vi "YKMW100 Write Com Register.vi"(0 "VISA session":refnum<visa-resource-name>="MW100", 2 "Semiphore":T1, 5 "Channel":string="C001", 7 "Value":string="000", 11 "error in (no error)":errorcluster) -> (4 "dup VISA session":refnum<visa-resource-name>="MW100", 15 "error out":errorcluster)   [LabVIEW 2009]
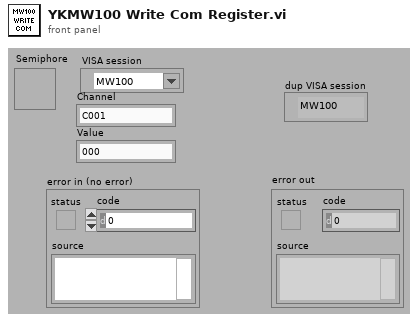
[diagram p1: front panel]
types:
  T1 = typedef "Semaphore RefNum" = refnum<k1>
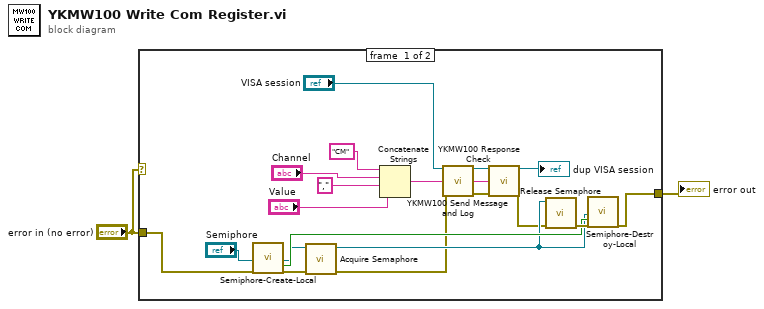
[diagram p0: block diagram]
diagram:
  n1 = case shown="No Error" "error in (no error)" {
    selector: "error in (no error)" -> [_ w23]
    tunnel: [w5 w23] -> w2
    tunnel: "error in (no error)" -> [w6 _]
    frame #0 {
      n2 = call "Semiphore-Create-Local.vi"("Semiphore"="Semiphore", "error in (no error)"=w6) -> ("semaphore"=w8:T1, "Local?"=w11:bool, "error out"=w9:errorcluster)  [unwired: 15 in]
      n3 = call <vilib>:"Acquire Semaphore.vi"("error in (no error)"=w9, "semaphore"=w8) -> ("error out"=w4:errorcluster, "semaphore out"=w10:T1)  [unwired: 3 in, 1 out]
      n4 = Concatenate Strings("CM" ("string"), "Channel", "," ("string"), "Value") -> (w13:string)
      n5 = call "YKMW100 Send Message and Log.vi"("VISA session"="VISA session", "Send Message (\"\")"=w13, "error in (no error)"=w4) -> ("dup VISA session"=w22:refnum<visa-resource-name>, "Read Buffer"=w20:string, "error out"=w21:errorcluster)  [unwired: 10 in]
      n6 = call "YKMW100 Response Check.vi"("VISA session"=w22, "Message In (\"\")"=w20, "error in (no error)"=w21) -> ("dup VISA session"=→"dup VISA session":refnum<visa-resource-name>, "error out"=w3:errorcluster)  [unwired: 8 in, 3 out]
      n7 = call <vilib>:"Release Semaphore.vi"("error in (no error)"=w3, "semaphore"=w10) -> ("error out"=w12:errorcluster)  [unwired: 4 in, 1 out]
      n8 = call "Semiphore-Destroy-Local.vi"("Semiphore"=w10, "Local?"=w11, "error in (no error)"=w12) -> ("error out"=w5:errorcluster)  [unwired: 16 in]
    }
    frame #1 {
    }
  }
  "error out" <- w2
